vi "Upload Register Log into Device.vi"(7 "Unit ID":string="A", 8 "error in (no error)":errorcluster, 10 "Run from \ninside of a VI?":bool, 11 "VISA Sesssion In":refnum<visa-resource-name>="COM4") -> (0 "error out":errorcluster, 1 "Confirmation Text":string, 2 "New Unit ID":string, 3 "VISA Session Out":refnum<visa-resource-name>)   [LabVIEW 2020]
doc: "Loads a text file log of register numbers and their corresponding values into LabVIEW, and writes all of the values into the corresponding Alicat registers."
uses:
  <vilib>/Utility/file.llb/Read From Spreadsheet File (DBL).vi
  <vilib>/Utility/file.llb/Read From Spreadsheet File (string).vi
panel:
  in  "Baud Rate":T1(ring)=enum."19200"
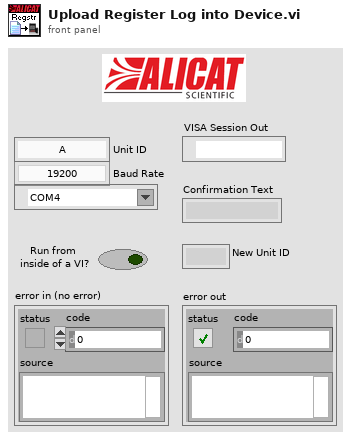
[diagram p1: front panel]
types:
  T1 = enum8{"2400", "9600", "19200", "38400", "57600", "115200", "Unknown"}
  T2 = cluster{"Unit ID":string, "Baud Rate":enum8{"2400", "9600", "19200", "38400", "57600", "115200", "Unknown"}, "VISA Sesssion In":refnum<visa-resource-name>}
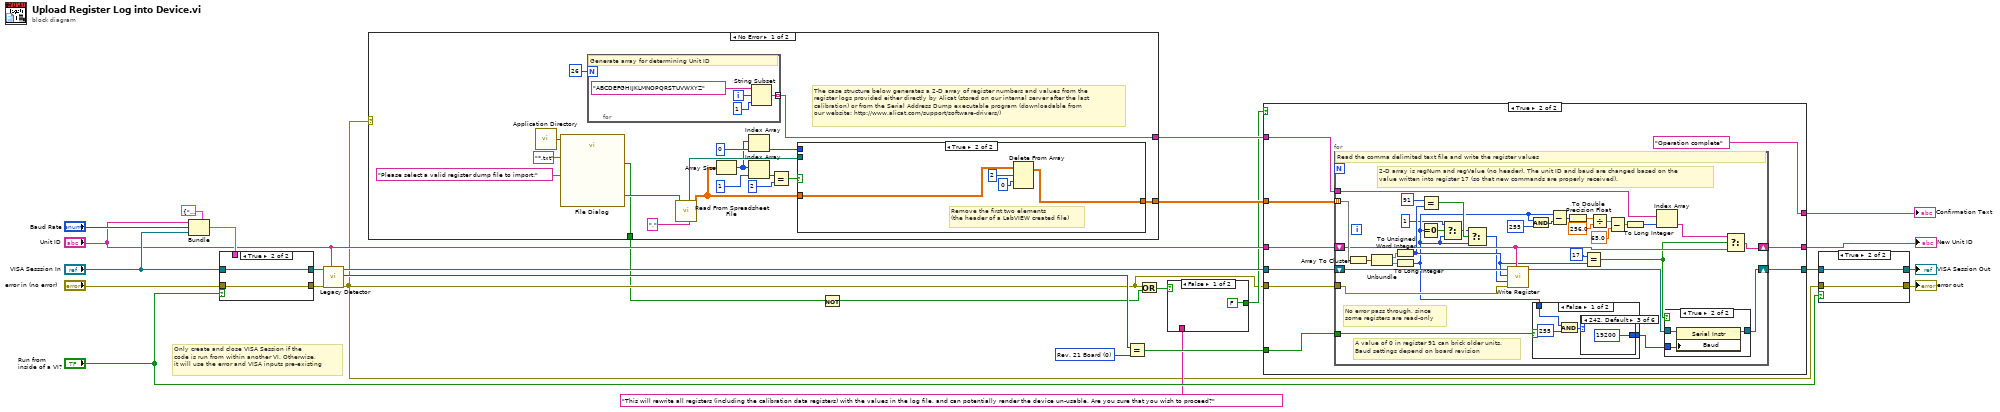
[diagram p0: block diagram]
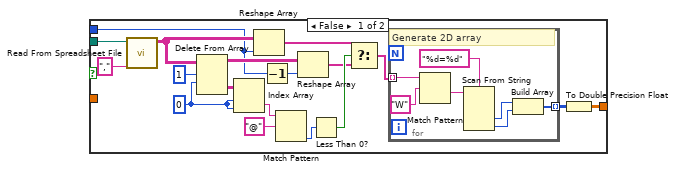
[diagram p2: hidden frame]
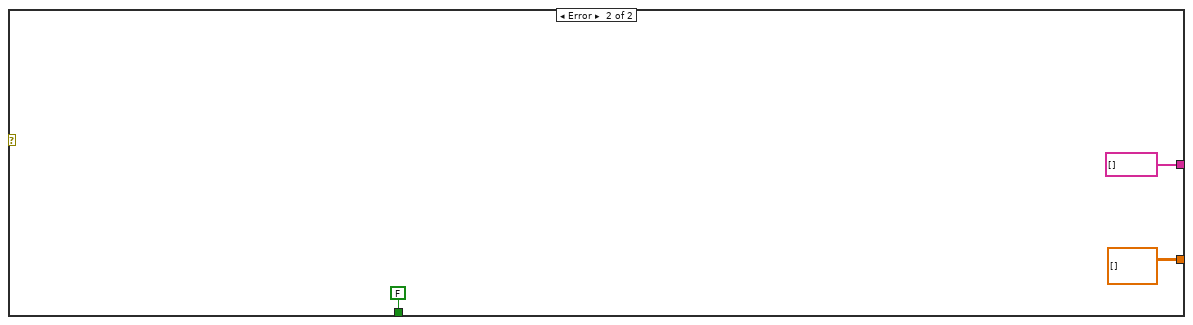
[diagram p3: hidden frame]
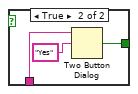
[diagram p4: hidden frame]
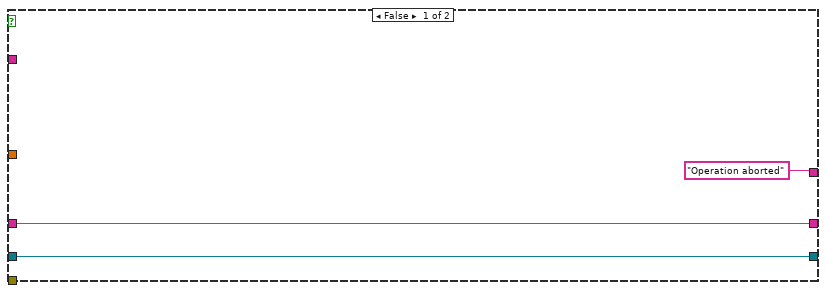
[diagram p5: hidden frame]
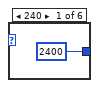
[diagram p6: hidden frame]
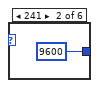
[diagram p7: hidden frame]
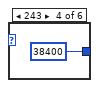
[diagram p8: hidden frame]
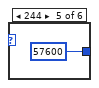
[diagram p9: hidden frame]
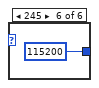
[diagram p10: hidden frame]
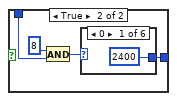
[diagram p11: hidden frame]
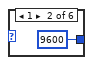
[diagram p12: hidden frame]
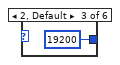
[diagram p13: hidden frame]
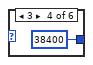
[diagram p14: hidden frame]
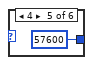
[diagram p15: hidden frame]
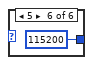
[diagram p16: hidden frame]
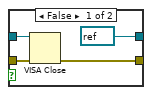
[diagram p18: hidden frame]
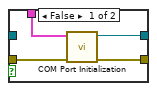
[diagram p19: hidden frame]
diagram:
  w10 = u8 0 items=["Rev. 21 Board", "Rev. 22 Board", "Rev. 23 Board"] ("Legacy Status")
  # "Only create and close VISA Session if the\ncode is run from within another VI. Otherwise,\nit will use the error and VISA inputs pre-existing"
  n1 = Bundle(cluster=T2 {"Unit ID"="A", "Baud Rate"=enum."19200", "VISA Sesssion In"="COM1"} ("Communication Settings"), "Unit ID"="Unit ID", "Baud Rate"="Baud Rate", "VISA Sesssion In"="VISA Sesssion In") -> (w15:T2)
  n2 = case shown="True" "Run from \ninside of a VI?" {
    tunnel: [w30 w32] -> w13
    tunnel: [w29 w31] -> w12
    tunnel: "error in (no error)" -> [w28 w32]
    tunnel: "VISA Sesssion In" -> [_ w31]
    tunnel: w15 -> [w27 _]
    frame False {
      n3 = call "COM Port Initialization.vi"("error in (no error)"=w28, "Communication Settings"=w27) -> ("error out"=w30:errorcluster, "VISA Session Out"=w29:refnum<visa-resource-name>)  [unwired: 8 in]
    }
    frame True {
    }
  }
  n4 = call "Legacy Detector.vi"("Unit ID (A)"="Unit ID", "error in"=w13, "VISA Session In"=w12) -> ("error out"=w3:errorcluster, "Legacy Status"=w9:u8, "VISA Session Out"=w14:refnum<visa-resource-name>)  [unwired: 6 in]
  n5 = case shown="No Error" w3 {
    tunnel: [w41 string[] []] -> w25
    tunnel: [w39 dbl[][] [] ("all rows")] -> w19
    tunnel: [w33 FALSE ("cancelled")] -> w2
    frame No Error {
      # "The case structure below generates a 2-D array of register numbers and values from the\nregister logs provided either directly by Alicat (stored on our internal server after the last\ncalibration) or from the Serial Address Dump executable program (downloadable from\nour website: http://www.alicat.com/support/software-drivers/)"
      n6 = call <vilib>:"Application Directory.vi"() -> ("Application Directory"=w49:path)
      n7 = call "File Dialog"("start path"=w49, "prompt"="Please select a valid register dump file to import:", "pattern (all files)"="*.txt") -> ("selected path"=w47:path, "cancelled"=w33:bool)  [unwired: 9 in, 2 out]
      n8 = for {
        N: 26 -> [_]
        tunnel: [w80] -> w41 mode=indexing
        i -> [w81]
        # "Generate array for determining Unit ID"
        n9 = String Subset(string="ABCDEFGHIJKLMNOPQRSTUVWXYZ", offset (0)=w81, length (rest)=1 ("length (rest)")) -> (substring=w80:string)
      }
      n10 = call-poly <vilib>:"Read From Spreadsheet File.vi"("delimiter (\\t)"="," ("delimiter (\\t)"), "file path (dialog if empty)"=w47) -> ("all rows"=w40:dbl[][], "new file path (Not A Path if cancelled)"=w37:path)  [unwired: 5 in, 3 out]
      n11 = Array Size(array=w40) -> (size(s)=w35:i32[])
      n12 = Index Array(array=w35, index=0) -> (element=w34:i32)
      n13 = Index Array(array=w35, index=1) -> (element=w45:i32)
      n14 = Equal?(x=w45, y=2) -> (x = y?=w38:bool)
      n15 = case shown="True" w38 {
        tunnel: [w51 w77] -> w39
        tunnel: w40 -> [_ w79]
        tunnel: w37 -> [w67 _]
        tunnel: w34 -> [w54 _]
        frame False {
          w62 = 0 ("index (row)")
          n16 = call-poly <vilib>:"Read From Spreadsheet File.vi"("delimiter (\\t)"="," ("delimiter (\\t)"), "file path (dialog if empty)"=w67) -> ("all rows"=w58:string[][])  [unwired: 5 in, 4 out]
          n17 = Delete From Array(array=w58, length=1, index (row)=w62) -> (deleted portion=w64:string[][], array with subset deleted=w55:string[][])  [unwired: 1 in]
          n18 = Index Array(array=w64, index (row)=w62, index (col)=w62) -> (element=w65:string)
          n19 = Reshape Array(w58, w54) -> (w57:string[])
          n20 = Decrement(x=w54) -> (x-1=w53:i32)
          n21 = Match Pattern(string=w65, regular expression="@") -> (offset past match=w61:i32)  [unwired: 1 in, 3 out]
          n22 = Reshape Array(w55, w53) -> (w56:string[])
          n23 = Less Than 0?(x=w61) -> (x < 0?=w60:bool)
          n24 = Select(t=w57, s=w60, f=w56) -> (s? t:f=w59:string[])
          n25 = for {
            tunnel: w59 -> [w74] mode=indexing
            tunnel: [w71] -> w52 mode=indexing
            # "Generate 2D array"
            n26 = Match Pattern(string=w74, regular expression="W") -> (after substring=w72:string)  [unwired: 1 in, 3 out]
            n27 = Scan From String(format string="%d=%d", input string=w72) -> (output 1=w69:i32, output 2=w70:i32)  [unwired: 4 in, 3 out]
            n28 = Build Array(w69, w70) -> (w71:i32[])
          }
          n29 = To Double Precision Float(number=w52) -> (double precision float=w51:dbl[][])
        }
        frame True {
          # "Remove the first two elements\n(the header of a LabVIEW created file)"
          n30 = Delete From Array(array=w79, length=2, index (row)=0) -> (array with subset deleted=w77:dbl[][])  [unwired: 1 in, 1 out]
        }
      }
    }
    frame Error {
    }
  }
  n31 = Not(x=w2) -> (.not. x?=w1:bool)
  n32 = Equal?(x=w9, y=w10) -> (x = y?=w8:bool)
  n33 = Or(x=w3, y=w1) -> (x .or. y?=w4:bool)
  n34 = case shown="False" w4 {
    tunnel: "This will rewrite all registers (including the calibration data registers) with the values in the log file, and can potentially render the device un-usable. Are you sure that you wish to proceed?" ("message") -> [_ w90]
    tunnel: [FALSE ("T button?") w88] -> w6
    frame False {
    }
    frame True {
      n35 = Two Button Dialog(message=w90, 2:"Yes" ("T button name (\"OK\")")) -> (T button?=w88:bool)  [unwired: 1 in]
    }
  }
  n36 = case shown="True" w6 {
    tunnel: [w91 w102] -> w26
    tunnel: w25 -> [_ w101]
    tunnel: [w92 w100] -> w24
    tunnel: w19 -> [_ w99]
    tunnel: w3 -> [_ w98]
    tunnel: w14 -> [w91 w97]
    tunnel: "Unit ID" -> [w92 w96]
    tunnel: w8 -> [_ w95]
    tunnel: ["Operation aborted" ("message") "Operation complete" ("message")] -> w5
    frame False {
    }
    frame True {
      n37 = for {
        tunnel: w99 -> [w135] mode=indexing
        shift-right: [w115] -> w102
        shift-left: w97 -> [w134]
        tunnel: w98 -> [w132]
        shift-right: [w131] -> w100
        shift-left: w96 -> [w133]
        tunnel: w101 -> [w130]
        tunnel: w95 -> [w111]
        # "A value of 0 in register 91 can brick older units.\nBaud settings depend on board revision"
        # "No error pass through, since\nsome registers are read-only"
        # "2-D array is regNum and regValue (no header). The unit ID and baud are changed based on the\nvalue written into register 17 (so that new commands are properly received)."
        # "Read the comma delimited text file and write the register values"
        n38 = Array To Cluster(array=w135) -> (cluster=w129:cluster{"all rows[0]":dbl, "all rows[1]":dbl})
        n39 = Unbundle(w129) -> ("all rows[0]"=w128:dbl, "all rows[1]"=w127:dbl)
        n40 = To Unsigned Word Integer(number=w128) -> (unsigned 16bit integer=w109:u16)
        n41 = To Long Integer(number=w127) -> (32bit integer=w104:i32)
        n42 = Equal To 0?(x=w104) -> (x = 0?=w110:bool)
        n43 = Equal?(x=u16 91, y=w109) -> (x = y?=w106:bool)
        n44 = Select(t=1, s=w110, f=w104) -> (s? t:f=w105:i32)
        n45 = Select(t=w105, s=w106, f=w104) -> (s? t:f=w107:i32)
        n46 = call "Write Register.vi"("Unit ID (A)"=w133, "error in"=w132, "Register Value"=w107, "Register address"=w109, "VISA Session In"=w134) -> ("VISA Session Out"=w116:refnum<visa-resource-name>)  [unwired: 4 in, 2 out]
        n47 = And(x=w104, y=255 ("32bit integer")) -> (x .and. y?=w113:i32)
        n48 = case shown="False" w111 {
          tunnel: [w139 w149] -> w112
          tunnel: w104 -> [w136 w146]
          frame False {
            n49 = And(x=w136, y=255 ("32bit integer")) -> (x .and. y?=w138:i32)
            n50 = case shown="242, Default" w138 {
              tunnel: [u32 2400 u32 9600 u32 19200 u32 38400 u32 57600 u32 115200] -> w139
              frame 240 {
              }
              frame 241 {
              }
              frame 242, Default {
              }
              frame 243 {
              }
              frame 244 {
              }
              frame 245 {
              }
            }
          }
          frame True {
            # "Baud rate changes"
            n51 = And(x=8 ("32bit integer"), y=w146) -> (x .and. y?=w147:i32)
            n52 = case shown="0" w147 {
              tunnel: [u32 2400 u32 9600 u32 19200 u32 38400 u32 57600 u32 115200] -> w149
              frame 0 {
              }
              frame 1 {
              }
              frame 2, Default {
              }
              frame 3 {
              }
              frame 4 {
              }
              frame 5 {
              }
            }
          }
        }
        n53 = Subtract(x=w104, y=w113) -> (x-y=w125:i32)
        n54 = To Double Precision Float(number=w125) -> (double precision float=w124:dbl)
        n55 = Equal?(x=u16 17 ("unsigned 16bit integer"), y=w109) -> (x = y?=w114:bool)
        n56 = Divide(x=w124, y=256.0) -> (x/y=w121:dbl)
        n57 = Subtract(x=w121, y=65.0) -> (x-y=w119:dbl)
        n58 = To Long Integer(number=w119) -> (32bit integer=w118:i32)
        n59 = Index Array(array=w130, index=w118) -> (element=w117:string)
        n60 = case shown="True" w114 {
          tunnel: w116 -> [w156 w159]
          tunnel: [w156 w158] -> w115
          tunnel: w112 -> [_ w157]
          frame False {
          }
          frame True {
            n61 = property class="Serial Instr"(reference=w159, "Baud"=w157) -> (reference out=w158:refnum<visa-resource-name>)  [unwired: 1 in, 1 out]
          }
        }
        n62 = Select(t=w117, s=w114, f=w133) -> (s? t:f=w131:string)
      }
    }
  }
  "New Unit ID" <- w24
  "Confirmation Text" <- w5
  n63 = case shown="True" "Run from \ninside of a VI?" {
    tunnel: w3 -> [w163 w165]
    tunnel: w26 -> [w162 w164]
    tunnel: [w161 w165] -> w21
    tunnel: [refnum<visa-resource-name> refnum ("VISA Session In") w164] -> w20
    frame False {
      n64 = VISA Close(VISA resource name=w162, error in (no error)=w163) -> (error out=w161:errorcluster)
    }
    frame True {
    }
  }
  "error out" <- w21
  "VISA Session Out" <- w20
